vi "read card.vi"() -> ()   [LabVIEW 2014]
uses:
  <vilib>/DAQmx/create/channels.llb/DAQmx Create Channel (AI-Voltage-Basic).vi
  <vilib>/DAQmx/configure/timing.llb/DAQmx Timing (Sample Clock).vi
  <vilib>/DAQmx/read.llb/DAQmx Read (Analog 1D DBL 1Chan NSamp).vi
panel:
  in  "Cluster":T1={"physical channels"="", "minimum value "=-5.0, "maximum value"=5.0, "rate"=1000.0} {"rate" format="%0.2f"; "maximum value" format="%0.2f"; "minimum value" format="%0.2f"}
  out "error out":errorcluster
  in  "stop":bool
  out "Waveform Chart":dbl[](graph)
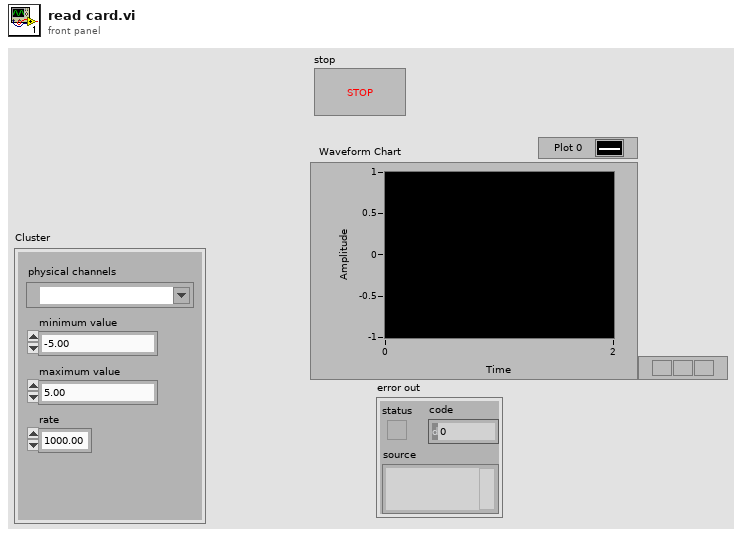
[diagram p1: front panel]
types:
  T1 = cluster{"physical channels":tag, "minimum value ":dbl, "maximum value":dbl, "rate":dbl}
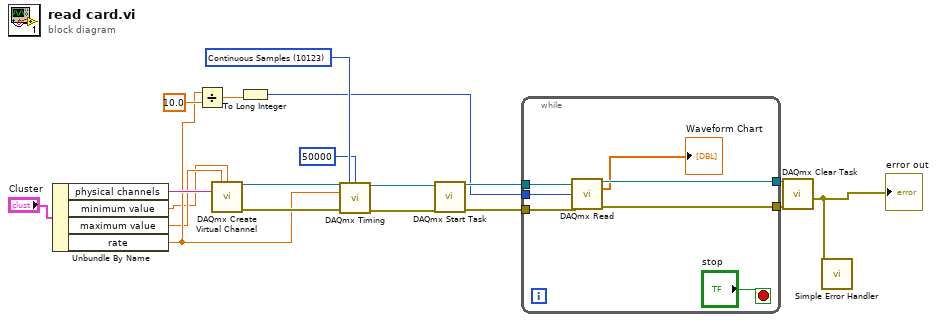
[diagram p0: block diagram]
diagram:
  w11 = 10123 items=["Finite Samples"=10178, "Continuous Samples"=10123, "Hardware Timed Single Point"=12522] ("sample mode")
  n1 = Unbundle By Name("Cluster") -> ("physical channels"=w8:tag, "minimum value"=w1:dbl, "maximum value"=w2:dbl, "rate"=w6:dbl)
  n2 = Divide(x=w6, y=10.0) -> (x/y=w5:dbl)
  n3 = call-poly <vilib>:"DAQmx Create Virtual Channel.vi"("maximum value"=w2, "minimum value"=w1, "physical channels"=w8) -> ("task out"=w17:refnum<k21>, "error out"=w12:errorcluster)  [unwired: 11 in]
  n4 = To Long Integer(number=w5) -> (32bit integer=w4:i32)
  n5 = call-poly <vilib>:"DAQmx Timing.vi"("task/channels in"=w17, "sample mode"=w11, "samples per channel"=50000, "rate"=w6, "error in"=w12) -> ("task out"=w18:refnum<k21>, "error out"=w19:errorcluster)  [unwired: 9 in]
  n6 = call <vilib>:"DAQmx Start Task.vi"("task/channels in"=w18, "error in"=w19) -> ("task out"=w14:refnum<k21>, "error out"=w16:errorcluster)  [unwired: 12 in]
  n7 = while {
    tunnel: w16 -> [w26]
    tunnel: [w25] -> w15
    tunnel: w14 -> [w24]
    tunnel: [w23] -> w13
    tunnel: w4 -> [w20]
    stop <- "stop" stop-if-true
    n8 = call-poly <vilib>:"DAQmx Read.vi"("task/channels in"=w24, "number of samples per channel"=w20, "error in"=w26) -> ("task out"=w23:refnum<k21>, "data"=→"Waveform Chart":dbl[], "error out"=w25:errorcluster)  [unwired: 10 in]
  }
  n9 = call <vilib>:"DAQmx Clear Task.vi"("task in"=w13, "error in"=w15) -> ("error out"=w10:errorcluster)  [unwired: 13 in]
  "error out" <- w10
  n10 = call <vilib>:"Simple Error Handler.vi"("error in (no error)"=w10) -> ()  [unwired: 4 in, 5 out]
